vi "Stop Core.vi"(10 "final error code":i32, 11 "uService Template in":refnum<class "Father of all uServices.lvclass">) -> (3 "uService Template out":refnum<class "Father of all uServices.lvclass">)   [LabVIEW 2026, in "TALOS.lvlib" / "Father of all uServices.lvlib" / "Father of all uServices.lvclass"]
doc: "(<B>Filename</B>: Actor Framework.lvlib:Actor.lvclass:Stop Core.vi)\n\nDefines what the actor does before it stops. Use the <B>final error code</B> input to determine whether the actor shut down in response to an error.\n\nBy default, this method passes the Stop message along to all auto-stop nested actors. A descendant class may override this method to define additional behavior, such as shutting down any processes the actor initiated in its override of the Actor Core method."
uses:
  Father of all uServices.lvclass
  Ancestor/Ancestor/Ancestor.lvclass
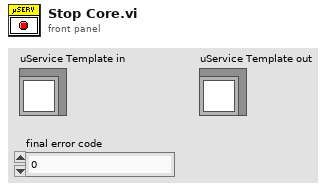
[diagram p1: front panel]
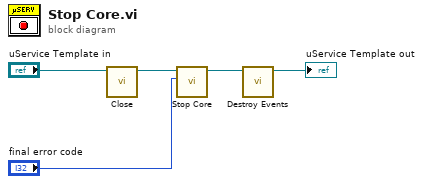
[diagram p0: block diagram]
diagram:
  n1 = call-dynamic "Close.vi"("uService Template in"="uService Template in") -> ("uService Template out"=w1:refnum<class "Father of all uServices.lvclass">)  [unwired: 9 in, 1 out]
  n2 = call-parent "Stop Core.vi"("final error code"="final error code", "Ancestor in"=w1) -> ("Ancestor out"=w4:refnum<class "Father of all uServices.lvclass">)  [unwired: 9 in]
  n3 = call-dynamic "Destroy Events.vi"("uService Template in"=w4) -> ("uService Template out"=→"uService Template out":refnum<class "Father of all uServices.lvclass">)  [unwired: 9 in, 1 out]
